vi "Update Configuration.vi"(8 "error in (no error)":errorcluster, 11 "CIFTemplateNode in":refnum<class "CIFCorePlugin.lvclass">) -> (0 "error out":errorcluster, 3 "CIFTemplateNode out":refnum<class "CIFCorePlugin.lvclass">)   [LabVIEW 2021, in "CIFCorePlugin.lvclass"]
uses:
  CIFCorePlugin.lvclass
  CIFCorePlugin.lvclass/CIFCorePlugin.ctl
  CIFUtilities/CIFOutOfBand/CIFOutOfBand.lvclass/CIFOutOfBand.ctl
  CIFCoreOOB/OOB_Rx/Private/Read Payload.vi
  Accessors/Timestamps/trash_Write ClockT0.vi
  CIFUtilities/CIFClocks/Core/Get Time.vi
  <vilib>/Utility/error.llb/Clear Errors.vi
  CIFUtilities/CIFOutOfBand/Accessors/Read Local OOB Data.vi
  CIFUtilities/CIFClocks/Time Conversion/LabVIEW Time to UTC Time.vi
  CIFUtilities/CIFClocks/SubVIs/Add Error.vi
  CIFCoreOOB/OOB_Rx/CIFCoreOOB_Rx.lvclass
  D:/dev/CIF-LVCore/src/CIFUtilities/CIFOutOfBand/CIFOutOfBand.lvclass
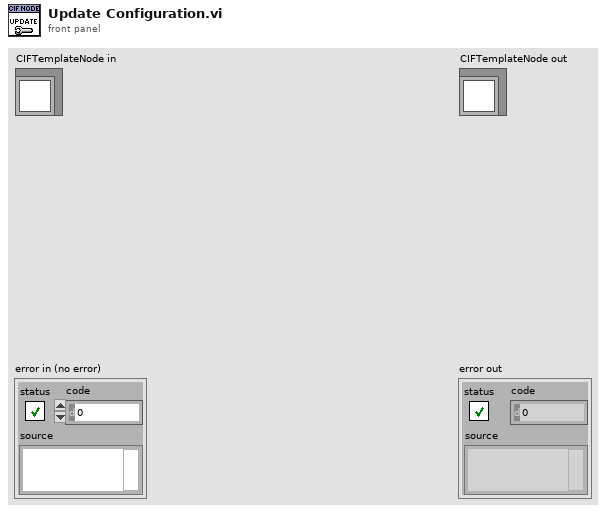
[diagram p1: front panel]
types:
  T1 = typedef "CIFCoreCommon.lvlib/Common Plugin Configuration.ctl" = cluster{"Period (s)":dbl, "Offset (us)":i32, "ClockID":u8, "Priority":i32, "Processor":i32}
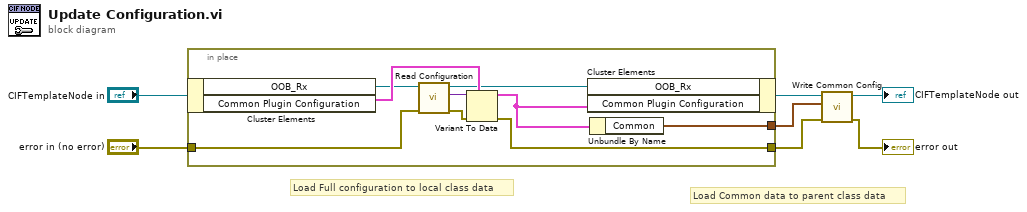
[diagram p0: block diagram]
diagram:
  # "Load Common data to parent class data"
  # "Load Full configuration to local class data"
  n1 = in-place {
    in-place-border: "error in (no error)" -> [w11]
    in-place-border: [w15] -> w3
    in-place-border: [w8] -> w4
    n2 = in-place-cluster #1("CIFTemplateNode in") -> ("OOB_Rx"=w14:refnum<class "CIFCoreOOB_Rx.lvclass">, "Common Plugin Configuration"=w16:cluster{"Common":T1})
    n3 = call "Read Configuration.vi"("error in"=w11, "CoreOOB_Rx in"=w14) -> ("error out"=w10:errorcluster, "Configuration Data"=w12:variant, "CoreOOB_Rx out"=w13:refnum<class "CIFCoreOOB_Rx.lvclass">)  [unwired: 7 in]
    n4 = Variant To Data(error in=w10, type=w16, Variant=w12) -> (data=w9:cluster{"Common":T1}, error out=w15:errorcluster)
    n5 = in-place-cluster #1("OOB_Rx"=w13, "Common Plugin Configuration"=w9) -> (w5:refnum<class "CIFCorePlugin.lvclass">)
    n6 = Unbundle By Name(w9) -> ("Common"=w8:T1)
  }
  n7 = call "Write Common Config.vi"("error in (no error)"=w3, "Common"=w4, "CIFTemplateNode in"=w5) -> ("error out"=→"error out":errorcluster, "CIFTemplateNode out"=→"CIFTemplateNode out":refnum<class "CIFCorePlugin.lvclass">)  [unwired: 7 in]
